vi "compute_statistics_data.vi"() -> ()   [LabVIEW 2020]
uses:
  StatisticsData.ctl
  ComputePhaseSet.lvclass
  WavefrontReconstructionMode.ctl
  HasoData.lvclass
  Phase.lvclass
  Pupil.lvclass
panel:
  out "Wavefront":sgl[][](graph)
  in  "Haso slopes file name":string="Data\\data_phase_computation.has"
  out "error out":errorcluster
  out "Statistics":T1
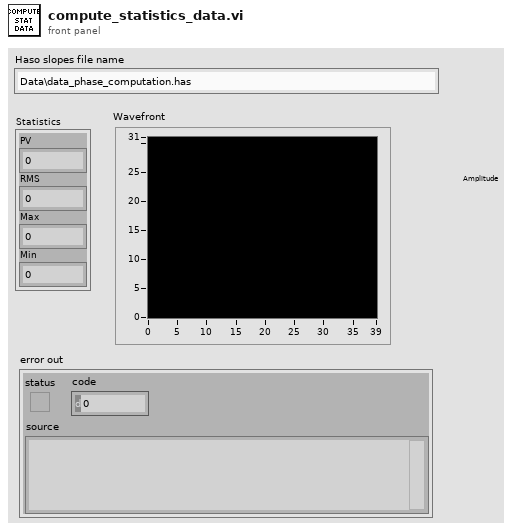
[diagram p1: front panel]
types:
  T1 = typedef "StatisticsData.ctl" = cluster{"PV":sgl, "RMS":dbl, "Max":sgl, "Min":sgl}
  T2 = typedef "WavefrontReconstructionMode.ctl" = enum16{"None", "Modal_Legendre", "Modal_Zernike", "Zonal", "Modal_Zonal_Zernike", "Modal_Zonal_Legendre"}
  T3 = typedef "Point2D.ctl" = cluster{"X":u32, "Y":u32}
  T4 = typedef "Point2Df.ctl" = cluster{"X":sgl, "Y":sgl}
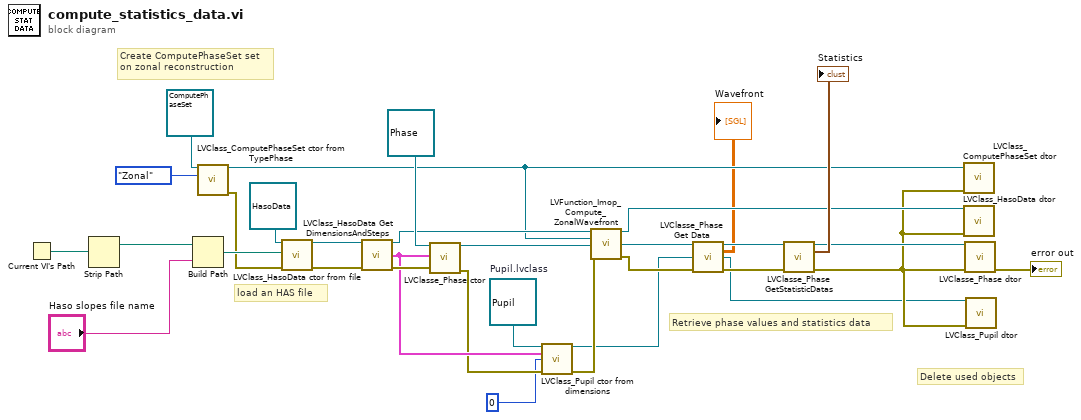
[diagram p0: block diagram]
diagram:
  w10 = refnum<class "Pupil.lvclass"> refnum  # Pupil.lvclass
  # "Delete used objects"
  # "Retrieve phase values and statistics data"
  # "Create ComputePhaseSet set\non zonal reconstruction"
  # "load an HAS file"
  n1 = Current VI's Path() -> (path=w19:path)
  n2 = Strip Path(path=w19) -> (stripped path=w16:path)  [unwired: 1 out]
  n3 = Build Path(base path=w16, name or relative path="Haso slopes file name") -> (appended path=w17:path)
  n4 = call "LVClass_ComputePhaseSet ctor from TypePhase.vi"("ComputePhaseSet (const)"=refnum<class "ComputePhaseSet.lvclass"> refnum ("ComputePhaseSet in"), "TypePhase"=WavefrontReconstructionMode."Zonal") -> ("ComputePhaseSet (new)"=w20:refnum<class "ComputePhaseSet.lvclass">, "error out"=w15:errorcluster)  [unwired: 12 in]
  n5 = call "LVClass_HasoData ctor from file.vi"("HasoData (const)"=refnum<class "HasoData.lvclass"> refnum ("HasoData in"), "HAS file path"=w17, "error in (no error)"=w15) -> ("HasoData (new)"=w29:refnum<class "HasoData.lvclass">, "error out"=w24:errorcluster)  [unwired: 11 in]
  n6 = call "LVClass_HasoData Get DimensionsAndSteps.vi"("HasoData in"=w29, "error in (no error)"=w24) -> ("HasoData out"=w27:refnum<class "HasoData.lvclass">, "Dimensions"=w9:cluster{"size":T3, "steps":T4}, "error out"=w25:errorcluster)  [unwired: 11 in]
  n7 = call "LVClasse_Phase ctor.vi"("Phase (const)"=refnum<class "Phase.lvclass"> refnum ("Phase in"), "Dimensions_um"=w9, "error in (no error)"=w25) -> ("Phase (new)"=w26:refnum<class "Phase.lvclass">, "error out"=w8:errorcluster)  [unwired: 11 in]
  n8 = call "LVClass_Pupil ctor from dimensions.vi"("Pupil (const)"=w10, "Dimensions_um"=w9, "value"=0, "error in (no error)"=w8) -> ("Pupil (new)"=w3:refnum<class "Pupil.lvclass">, "error out"=w6:errorcluster)  [unwired: 10 in]
  n9 = call "LVFunction_Imop_Compute_ZonalWavefront.vi"("HasoData.lvclass"=w27, "ComputePhaseSet.lvclass"=w20, "Phase"=w26, "error constant"=w6) -> ("HasoData.lvclass (dup)"=w21:refnum<class "HasoData.lvclass">, "Phase"=w14:refnum<class "Phase.lvclass">, "error out"=w5:errorcluster)  [unwired: 8 in, 1 out]
  n10 = call "LVClasse_Phase Get Data.vi"("Phase in"=w14, "Pupil"=w3, "error in (no error)"=w5) -> ("Phase out"=w13:refnum<class "Phase.lvclass">, "data"=→"Wavefront":sgl[][], "Pupil (dup)"=w2:refnum<class "Pupil.lvclass">, "error out"=w12:errorcluster)  [unwired: 9 in]
  n11 = call "LVClasse_Phase GetStatisticDatas.vi"("Phase in"=w13, "error in (no error)"=w12) -> ("Phase out"=w22:refnum<class "Phase.lvclass">, "StatisticsData"=→"Statistics":T1, "error out"=w4:errorcluster)  [unwired: 11 in]
  n12 = call "LVClass_ComputePhaseSet dtor.vi"("ComputePhaseSet in"=w20, "error in (no error)"=w4) -> ()  [unwired: 12 in, 2 out]
  n13 = call "LVClass_HasoData dtor.vi"("HasoData in"=w21, "error in (no error)"=w4) -> ()  [unwired: 12 in, 2 out]
  n14 = call "LVClasse_Phase dtor.vi"("Phase in"=w22, "error in (no error)"=w4) -> ("error out"=→"error out":errorcluster)  [unwired: 12 in, 1 out]
  n15 = call "LVClass_Pupil dtor.vi"("Pupil in"=w2, "error in (no error)"=w4) -> ()  [unwired: 12 in, 2 out]
